vi "sandbox.vi"() -> ()   [LabVIEW 2021]
panel:
  out "nearest integer value":i32
  out "x rotated left by y 3":u64=12302652056653603379 format="%.0x"
  out "x rotated left by y 2":u64=12302652056653603379 format="%.0x"
  out "x rotated left by y":u64 format="%.0x"
  out "x << y 3":i32
  out "x*y":i32
  out "x << y 2":i16
  out "floor(x/y) 2":i16
  out "x/y 2":dbl
  out "x << y":i16
  out "floor(x/y)":i16
  out "x/y":dbl
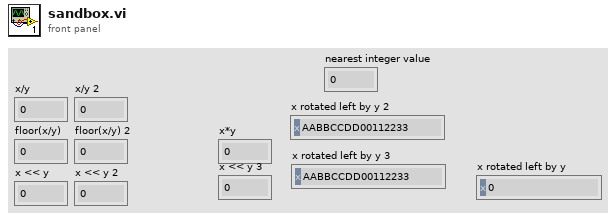
[diagram p1: front panel]
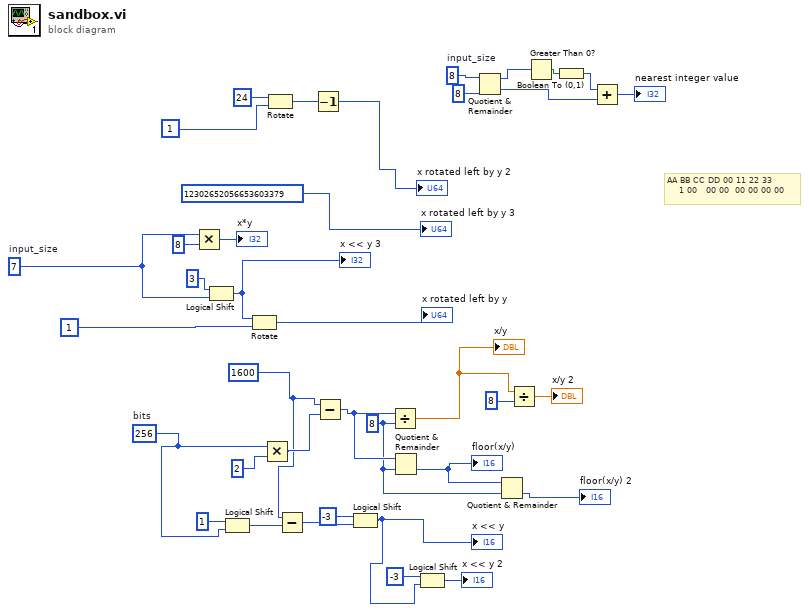
[diagram p0: block diagram]
diagram:
  w6 = 8  # input_size
  w17 = 7  # input_size
  w24 = i16 8 ("y")
  w31 = i16 1600
  w34 = i16 256  # bits
  # "AA BB CC DD 00 11 22 33\n    1 00   00 00  00 00 00 00"
  n1 = Multiply(x=w17, y=8) -> (x*y=→"x*y":i32)
  n2 = Logical Shift(y=i16 3, x=w17) -> (x << y=w14:i32)
  "x << y 3" <- w14
  n3 = Logical Shift(y=i16 1, x=w34) -> (x << y=w32:i16)
  n4 = Rotate(1:u64 1 ("y"), 2:w14) -> (0:→"x rotated left by y":u64)
  n5 = Multiply(x=w34, y=i16 2) -> (x*y=w36:i16)
  n6 = Rotate(1:u64 1 ("x rotated left by y"), 2:i16 24 ("y")) -> (0:w12:u64)
  n7 = Subtract(x=w31, y=w32) -> (x-y=w30:i16)
  n8 = Decrement(x=w12) -> (x-1=→"x rotated left by y 2":u64)
  n9 = Subtract(x=w31, y=w36) -> (x-y=w35:i16)
  n10 = Logical Shift(y=i16 -3, x=w30) -> (x << y=w21:i16)
  "x << y" <- w21
  n11 = Divide(x=w35, y=w24) -> (x/y=w27:dbl)
  "x/y" <- w27
  n12 = Quotient & Remainder(x=w35, y=w24) -> (floor(x/y)=w25:i16)  [unwired: 1 out]
  "floor(x/y)" <- w25
  n13 = Logical Shift(y=i16 -3, x=w21) -> (x << y=→"x << y 2":i16)
  n14 = Quotient & Remainder(x=w6, y=8) -> (x-y*floor(x/y)=w3:i32, floor(x/y)=w7:i32)
  n15 = Quotient & Remainder(x=w25, y=w24) -> (floor(x/y)=→"floor(x/y) 2":i16)  [unwired: 1 out]
  n16 = Divide(x=w27, y=i16 8) -> (x/y=→"x/y 2":dbl)
  n17 = Greater Than 0?(x=w3) -> (x > 0?=w2:bool)
  n18 = Boolean To (0,1)(Boolean=w2) -> (0, 1=w1:i16)
  n19 = Add(x=w1, y=w7) -> (x+y=→"nearest integer value":i32)
  "x rotated left by y 3" <- u64 12302652056653603379 ("x rotated left by y")
